vi "CreateNewWizard_GetWeight.vi"(11 "Wizard":T1) -> (3 "Weight":i32)   [LabVIEW 2023, in "Add Async Methods Actor.lvlib"]
uses:
  Add Async Methods Actor.lvlib
  <resource>/Framework/Providers/API/ItemRef.ctl
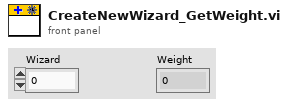
[diagram p1: front panel]
types:
  T1 = typedef "ItemRef.ctl" = u64
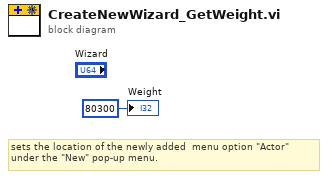
[diagram p0: block diagram]
diagram:
  # "sets the location of the newly added  menu option \"Actor\"\nunder the \"New\" pop-up menu."
  "Weight" <- 80300 ("Weight")
